vi "SDT_MeasureInfoBlockToSPCdata.vi"(11 "MeasureInfo":T1[](array[typedef]) {"MeasStopInfo"."flags" format="x%x"}) -> (2 "SPCdata":T11[](array[typedef]))   [LabVIEW 2019]
doc: "This VI is a SubVI to SDT_WriteFile.vi. It populates the arrays of MeasureInfos cluster and generates strings ready to be written to file. \nFor a description of the *.sdt file format see: SPC_data_file_structure.h\n\ninfo@becker-hickl.com"
uses:
  SPC_Controls/SPCdata.ctl
  SPC_Controls/MeasureInfo.ctl
  SPC_Controls/MeasureInfo_PartB.ctl
  SPC_Controls/MeasStopInfo.ctl
  SPC_Controls/MeasFCSInfo.ctl
  SPC_Controls/MeasureInfo_PartE.ctl
  SPC_Controls/MeasHISTInfo.ctl
  SPC_Controls/HISTInfoExt.ctl
  SPC_Controls/MeasureInfo_PartI.ctl
  SPC_Controls/MeasureInfo_PartK.ctl
  SPC_Controls/MeasureInfo_PartM.ctl
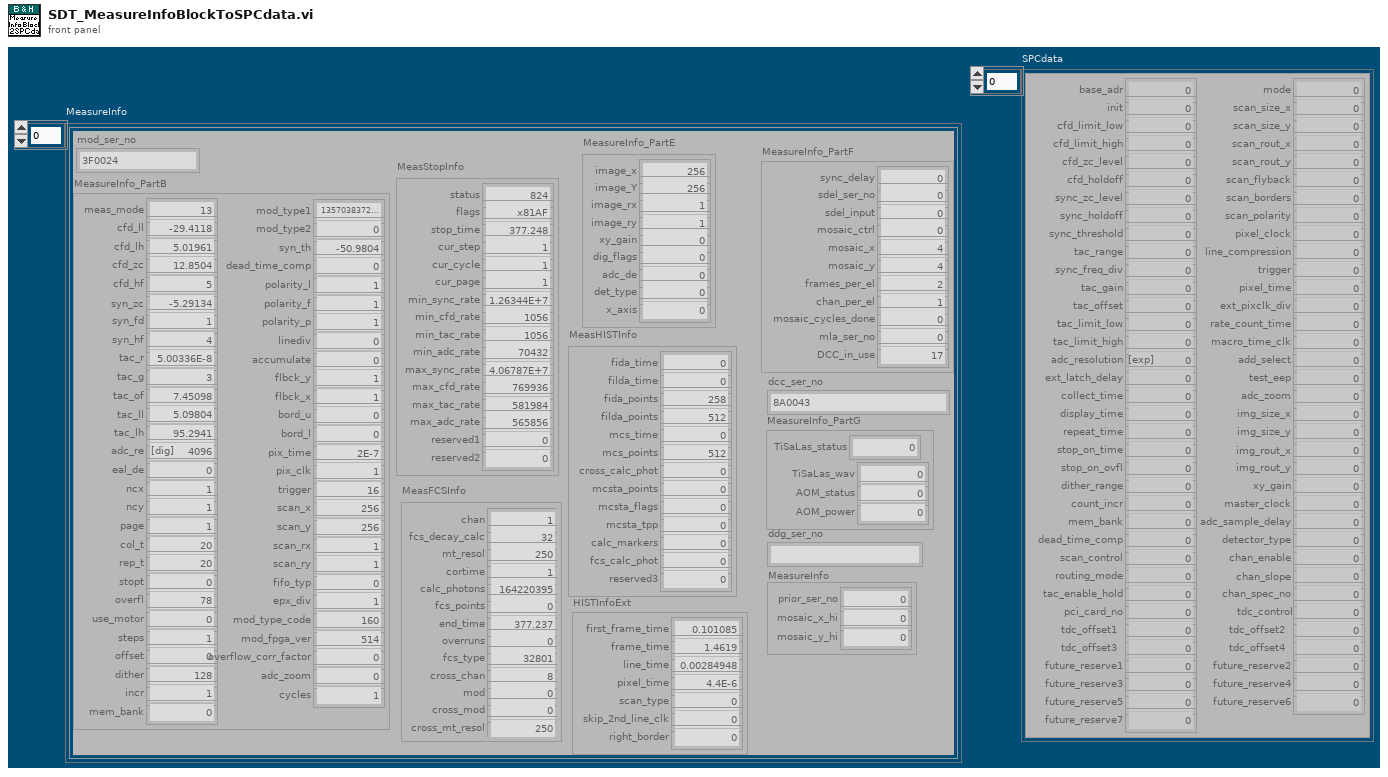
[diagram p1: front panel]
types:
  T1 = typedef "MeasureInfo.ctl" = cluster{"mod_ser_no":string, "MeasureInfo_PartB":T2, "MeasStopInfo":T3, "MeasFCSInfo":T4, "MeasureInfo_PartE":T5, "MeasHISTInfo":T6, "HISTInfoExt":T7, "MeasureInfo_PartF":T8, "dcc_ser_no":string, "MeasureInfo_PartG":T9, "ddg_ser_no":string, "MeasureInfo":T10}
  T2 = typedef "MeasureInfo_PartB.ctl" = cluster{"meas_mode":i16, "cfd_ll":sgl, "cfd_lh":sgl, "cfd_zc":sgl, "cfd_hf":sgl, "syn_zc":sgl, "syn_fd":i16, "syn_hf":sgl, "tac_r":sgl, "tac_g":i16, "tac_of":sgl, "tac_ll":sgl, "tac_lh":sgl, "adc_re":i16, "eal_de":i16, "ncx":i16, "ncy":i16, "page":u16, "col_t":sgl, "rep_t":sgl, "stopt":i16, "overfl":i8, "use_motor":i16, "steps":u16, "offset":sgl, "dither":i16, "incr":i16, "mem_bank":i16, "mod_type1":u64, "mod_type2":u64, "syn_th":sgl, "dead_time_comp":i16, "polarity_l":i16, "polarity_f":i16, "polarity_p":i16, "linediv":i16, "accumulate":i16, "flbck_y":i32, "flbck_x":i32, "bord_u":i32, "bord_l":i32, "pix_time":sgl, "pix_clk":i16, "trigger":i16, "scan_x":i32, "scan_y":i32, "scan_rx":i32, "scan_ry":i32, "fifo_typ":i16, "epx_div":i32, "mod_type_code":u16, "mod_fpga_ver":u16, "overflow_corr_factor":sgl, "adc_zoom":i32, "cycles":i32}
  T3 = typedef "MeasStopInfo.ctl" = cluster{"status":u16, "flags":u16, "stop_time":sgl, "cur_step":i32, "cur_cycle":i32, "cur_page":i32, "min_sync_rate":sgl, "min_cfd_rate":sgl, "min_tac_rate":sgl, "min_adc_rate":sgl, "max_sync_rate":sgl, "max_cfd_rate":sgl, "max_tac_rate":sgl, "max_adc_rate":sgl, "reserved1":i32, "reserved2":sgl}
  T4 = typedef "MeasFCSInfo.ctl" = cluster{"chan":u16, "fcs_decay_calc":u16, "mt_resol":u32, "cortime":sgl, "calc_photons":u32, "fcs_points":i32, "end_time":sgl, "overruns":u16, "fcs_type":u16, "cross_chan":u16, "mod":u16, "cross_mod":u16, "cross_mt_resol":u32}
  T5 = typedef "MeasureInfo_PartE.ctl" = cluster{"image_x":i32, "image_Y":i32, "image_rx":i32, "image_ry":i32, "xy_gain":i16, "dig_flags":i16, "adc_de":i16, "det_type":i16, "x_axis":i16}
  T6 = typedef "MeasHISTInfo.ctl" = cluster{"fida_time":sgl, "filda_time":sgl, "fida_points":i32, "filda_points":i32, "mcs_time":sgl, "mcs_points":i32, "cross_calc_phot":u32, "mcsta_points":u16, "mcsta_flags":u16, "mcsta_tpp":u32, "calc_markers":u32, "fcs_calc_phot":u32, "reserved3":u32}
  T7 = typedef "HISTInfoExt.ctl" = cluster{"first_frame_time":sgl, "frame_time":sgl, "line_time":sgl, "pixel_time":sgl, "scan_type":i16, "skip_2nd_line_clk":i16, "right_border":u32}
  T8 = typedef "MeasureInfo_PartI.ctl" = cluster{"sync_delay":sgl, "sdel_ser_no":u16, "sdel_input":i8, "mosaic_ctrl":i8, "mosaic_x":u8, "mosaic_y":u8, "frames_per_el":i16, "chan_per_el":i16, "mosaic_cycles_done":i32, "mla_ser_no":u16, "DCC_in_use":u8}
  T9 = typedef "MeasureInfo_PartK.ctl" = cluster{"TiSaLas_status":u16, "TiSaLas_wav":u16, "AOM_status":u8, "AOM_power":u8}
  T10 = typedef "MeasureInfo_PartM.ctl" = cluster{"prior_ser_no":i32, "mosaic_x_hi":u8, "mosaic_y_hi":u8}
  T11 = typedef "SPCdata.ctl" = cluster{"base_adr":u16, "init":i16, "cfd_limit_low":sgl, "cfd_limit_high":sgl, "cfd_zc_level":sgl, "cfd_holdoff":sgl, "sync_zc_level":sgl, "sync_holdoff":sgl, "sync_threshold":sgl, "tac_range":sgl, "sync_freq_div":i16, "tac_gain":i16, "tac_offset":sgl, "tac_limit_low":sgl, "tac_limit_high":sgl, "adc_resolution":i16, "ext_latch_delay":i16, "collect_time":sgl, "display_time":sgl, "repeat_time":sgl, "stop_on_time":i16, "stop_on_ovfl":i16, "dither_range":i16, "count_incr":i16, "mem_bank":i16, "dead_time_comp":i16, "scan_control":u16, "routing_mode":u16, "tac_enable_hold":sgl, "pci_card_no":i16, "mode":u16, "scan_size_x":u32, "scan_size_y":u32, "scan_rout_x":u32, "scan_rout_y":u32, "scan_flyback":u32, "scan_borders":u32, "scan_polarity":u16, "pixel_clock":u16, "line_compression":u16, "trigger":u16, "pixel_time":sgl, "ext_pixclk_div":u32, "rate_count_time":sgl, "macro_time_clk":i16, "add_select":i16, "test_eep":i16, "adc_zoom":i16, "img_size_x":u32, "img_size_y":u32, "img_rout_x":u32, "img_rout_y":u32, "xy_gain":i16, "master_clock":i16, "adc_sample_delay":i16, "detector_type":i16, "chan_enable":u32, "chan_slope":u32, "chan_spec_no":u32, "tdc_control":u32, "tdc_offset1":sgl, "tdc_offset2":sgl, "tdc_offset3":sgl, "tdc_offset4":sgl, "future_reserve1":u64, "future_reserve2":u64, "future_reserve3":u64, "future_reserve4":u64, "future_reserve5":u64, "future_reserve6":u64, "future_reserve7":u64}
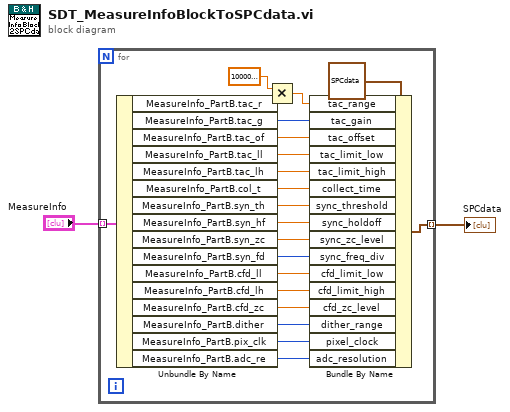
[diagram p0: block diagram]
diagram:
  n1 = for {
    tunnel: "MeasureInfo" -> [w23] mode=indexing
    tunnel: [w6] -> w1 mode=indexing
    n2 = Unbundle By Name(w23) -> ("MeasureInfo_PartB.tac_r"=w4:sgl, "MeasureInfo_PartB.tac_g"=w9:i16, "MeasureInfo_PartB.tac_of"=w10:sgl, "MeasureInfo_PartB.tac_ll"=w11:sgl, "MeasureInfo_PartB.tac_lh"=w12:sgl, "MeasureInfo_PartB.col_t"=w13:sgl, "MeasureInfo_PartB.syn_th"=w14:sgl, "MeasureInfo_PartB.syn_hf"=w15:sgl, "MeasureInfo_PartB.syn_zc"=w16:sgl, "MeasureInfo_PartB.syn_fd"=w17:i16, "MeasureInfo_PartB.cfd_ll"=w18:sgl, "MeasureInfo_PartB.cfd_lh"=w19:sgl, "MeasureInfo_PartB.cfd_zc"=w20:sgl, "MeasureInfo_PartB.dither"=w21:i16, "MeasureInfo_PartB.pix_clk"=w22:i16, "MeasureInfo_PartB.adc_re"=w3:i16)
    n3 = Multiply(x=sgl 1000000000.0 ("y"), y=w4) -> (x*y=w5:sgl)
    n4 = Bundle By Name(cluster=T11 {"base_adr"=0, "init"=0, "cfd_limit_low"=0.0, "cfd_limit_high"=0.0, "cfd_zc_level"=0.0, "cfd_holdoff"=0.0, "sync_zc_level"=0.0, "sync_holdoff"=0.0, "sync_threshold"=0.0, "tac_range"=0.0, "sync_freq_div"=0, "tac_gain"=0, "tac_offset"=0.0, "tac_limit_low"=0.0, "tac_limit_high"=0.0, "adc_resolution"=0, "ext_latch_delay"=0, "collect_time"=0.0, "display_time"=0.0, "repeat_time"=0.0, "stop_on_time"=0, "stop_on_ovfl"=0, "dither_range"=0, "count_incr"=0, "mem_bank"=0, "dead_time_comp"=0, "scan_control"=0, "routing_mode"=0, "tac_enable_hold"=0.0, "pci_card_no"=0, "mode"=0, "scan_size_x"=0, "scan_size_y"=0, "scan_rout_x"=0, "scan_rout_y"=0, "scan_flyback"=0, "scan_borders"=0, "scan_polarity"=0, "pixel_clock"=0, "line_compression"=0, "trigger"=0, "pixel_time"=0.0, "ext_pixclk_div"=0, "rate_count_time"=0.0, "macro_time_clk"=0, "add_select"=0, "test_eep"=0, "adc_zoom"=0, "img_size_x"=0, "img_size_y"=0, "img_rout_x"=0, "img_rout_y"=0, "xy_gain"=0, "master_clock"=0, "adc_sample_delay"=0, "detector_type"=0, "chan_enable"=0, "chan_slope"=0, "chan_spec_no"=0, "tdc_control"=0, "tdc_offset1"=0.0, "tdc_offset2"=0.0, "tdc_offset3"=0.0, "tdc_offset4"=0.0, "future_reserve1"=0, "future_reserve2"=0, "future_reserve3"=0, "future_reserve4"=0, "future_reserve5"=0, "future_reserve6"=0, "future_reserve7"=0} ("SPCdata"), "tac_range"=w5, "tac_gain"=w9, "tac_offset"=w10, "tac_limit_low"=w11, "tac_limit_high"=w12, "collect_time"=w13, "sync_threshold"=w14, "sync_holdoff"=w15, "sync_zc_level"=w16, "sync_freq_div"=w17, "cfd_limit_low"=w18, "cfd_limit_high"=w19, "cfd_zc_level"=w20, "dither_range"=w21, "pixel_clock"=w22, "adc_resolution"=w3) -> (w6:T11)
  }
  "SPCdata" <- w1
